vi "Main.vi"   [LabVIEW 2021]
uses:
  Library/Library.lvlib
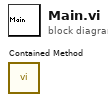
[diagram p0: block diagram]
diagram:
  n1 = call "Contained Method.vi"() -> ()  [unwired: 12 in]
